vi "Lift Wrapper.vi"(10 "Lift down":bool, 11 "Lift up":bool) -> ()   [LabVIEW 2014]
uses:
  Precreated VIs/Robot Global Data.vi
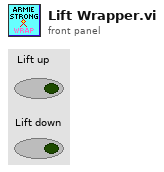
[diagram p1: front panel]
types:
  T1 = cluster{"Distance":dbl, "Rate":dbl, "Direction":bool, "Stopped":bool}
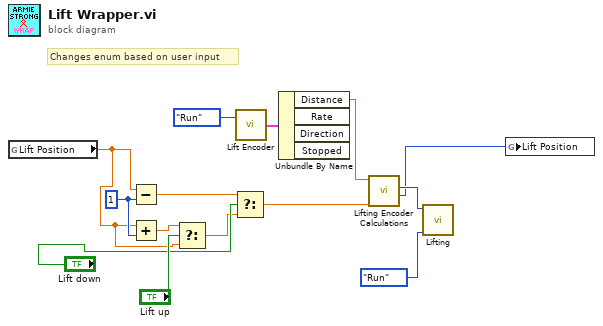
[diagram p0: block diagram]
diagram:
  w3 = 1
  # "Changes enum based on user input"
  n1 = global read "Robot Global Data.vi" "Lift Position"() -> (w2:dbl)
  n2 = Subtract(x=w2, y=w3) -> (x-y=w5:dbl)
  n3 = Add(x=w2, y=w3) -> (x+y=w6:dbl)
  n4 = Select(t=w6, s="Lift up", f=w2) -> (s? t:f=w4:dbl)
  n5 = Select(t=w5, s="Lift down", f=w4) -> (s? t:f=w7:dbl)
  n6 = call "Lift Encoder.vi"("Mode"=enum8{"Start", "Run", "Finish"}."Run") -> ("Lift Encoder"=w13:T1)  [unwired: 1 in]
  n7 = Unbundle By Name(w13) -> ("Distance"=w12:dbl)  [unwired: 3 out]
  n8 = call "Lifting Encoder Calculations.vi"("Position"=w7, "distance traveled"=w12) -> ("Current position"=w1:i32, "Direction"=w11:enum16{"stop", "up", "down"})  [unwired: 7 in]
  n9 = call "Lifting.vi"("Direction"=w11, "Mode"=enum8{"Start", "Run", "Finish"}."Run") -> ()  [unwired: 4 in]
  n10 = global write "Robot Global Data.vi" "Lift Position"(w1) -> ()
